vi "ADIS16470 Open.vi"(7 "Buffer Size (0)":u32, 8 "error in":errorcluster, 9 "Initial Calibration Time (4s)":dbl=4.0, 10 "Sychronous Process VI":T1, 11 "Hardware Config":T3={"SPI Clock Rate (Hz)"=2000000.0, "IMU SPI Mode (3)"=enum."Mode 3 (Clk Idle High,Sample on Trailing)", "IMU Reset Pin"=enum."SPI Port CS2", "IMU SPI Bus"=enum."SPI On-Board, CS0", "IMU Data Ready Pin"=enum."SPI Port CS1", "Stall Config"={"Pow2BytesPerRead"=1, "StallTicks"=1000, "CsToSclkTicks"=5}}) -> (0 "error out":errorcluster, 3 "ADIS16470DevRef":T2={"DevStatus"={"status"=FALSE, "code"=0, "source"=""}, "Hardware Config"={"SPI Clock Rate (Hz)"=1000000.0, "IMU SPI Mode (3)"=enum."Mode 3 (Clk Idle High,Sample on Trailing)", "IMU Reset Pin"=enum."SPI Port CS2", "IMU SPI Bus"=enum."SPI On-Board, CS0", "IMU Data Ready Pin"=enum."SPI Port CS1", "Stall Config"={"Pow2BytesPerRead"=255, "StallTicks"=640, "CsToSclkTicks"=5}}, "Calibration Complete"=refnum, "Status Reference"=refnum, "Data Reference"=refnum, "Sychronous Process VI"=refnum, "Cmd FIFO"=refnum, "Source"={"DevStatus"={"status"=FALSE, "code"=0, "source"=""}, "AnalogTriggerMode?"=FALSE, "DigitalMode"={"DIO Channel"=enum."Disabled"}, "AnalogTriggerMode"={"AnalogTriggerIndex"=enum."Trig 0", "OutputType"=enum."InWindow"}}, "Data FIFO"=refnum, "Calibration Time (ms)"=5, "Data Reference"=refnum})   [LabVIEW 2025]
doc: "Open and initialize a session for the ADI 16470 IMU. This calibrates, and then integrates X, Y, and Z angles. Acceleration and other IMU values are not currently surfaced, but are accessible if added to the API. It is advised that you have the robot stationary while being calibrated."
uses:
  <vilib>/Rock Robotics/WPI/ThirdParty/ADI/ADIS16470/Typedef/ADIS16470 Hardware Configuration.ctl
  <vilib>/Rock Robotics/WPI/SPI/WPI_SPIMode.ctl
  <vilib>/Rock Robotics/SystemInterfaces/DIO/FPGA_DIOChannel.ctl
  <vilib>/Rock Robotics/SystemInterfaces/spilib/spi_bus.ctl
  <vilib>/Rock Robotics/WPI/ThirdParty/ADI/ADIS16470/Typedef/ADIS16470 Device Reference.ctl
  <vilib>/Rock Robotics/WPI/ThirdParty/ADI/ADIS16470/Typedef/ADIS16470 Status.ctl
  <vilib>/Rock Robotics/WPI/ThirdParty/ADI/ADIS16470/Typedef/ADIS16470 Data.ctl
  <vilib>/Rock Robotics/WPI/ThirdParty/ADI/ADIS16470/Typedef/ADIS16470 Process.ctl
  <vilib>/Rock Robotics/WPI/ThirdParty/ADI/ADIS16470/Typedef/ADIS16470 Command Type.ctl
  <vilib>/Rock Robotics/SystemInterfaces/CounterEncoderSourceConvertion/FPGA_CounterEncoderSourceConvertionLVSourceType.ctl
  <vilib>/Rock Robotics/SystemInterfaces/DIO/FPGA_DIODigitalSourceChannel.ctl
  <vilib>/Rock Robotics/SystemInterfaces/AnalogTrigger/FPGA_AnalogTriggerIndex.ctl
  <vilib>/Rock Robotics/SystemInterfaces/AnalogTrigger/FPGA_AnalogTriggerOutType.ctl
  <vilib>/Rock Robotics/SystemInterfaces/NetworkCommunication/NetComm_UsageReport_ResourceType.ctl
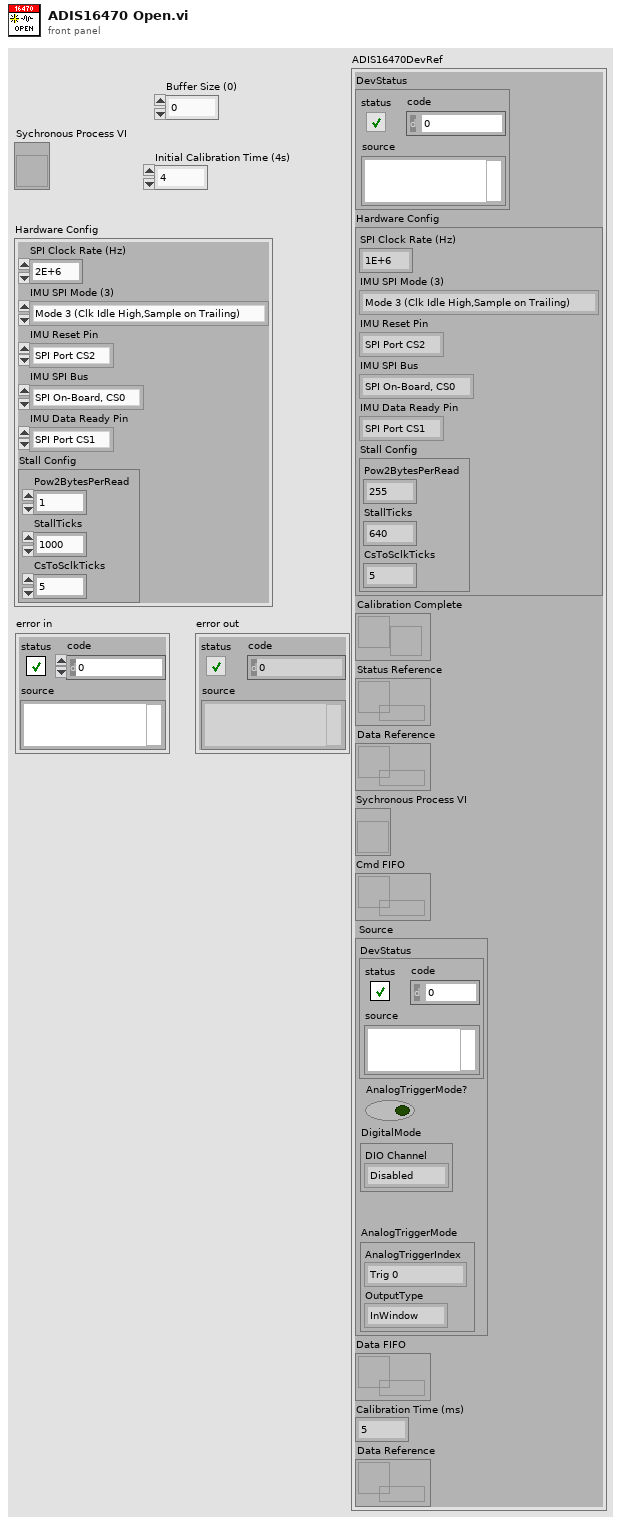
[diagram p1: front panel]
types:
  T1 = typedef "ADIS16470 Process.ctl" = refnum<vi>
  T2 = typedef "ADIS16470 Device Reference.ctl" = cluster{"DevStatus":errorcluster, "Hardware Config":T3, "Calibration Complete":refnum<notifier>, "Status Reference":refnum<data-value>, "Data Reference":refnum<data-value>, "Sychronous Process VI":T1, "Cmd FIFO":refnum<k33>, "Source":T7, "Data FIFO":refnum<k33>, "Calibration Time (ms)":u32, "Data Reference":refnum<data-value>}
  T3 = typedef "ADIS16470 Hardware Configuration.ctl" = cluster{"SPI Clock Rate (Hz)":dbl, "IMU SPI Mode (3)":T4, "IMU Reset Pin":T5, "IMU SPI Bus":T6, "IMU Data Ready Pin":T5, "Stall Config":cluster{"Pow2BytesPerRead":u8, "StallTicks":u16, "CsToSclkTicks":u8}}
  T4 = typedef "WPI_SPIMode.ctl" = enum16{"Mode 0 (Clk Idle Low,Sample on Leading)", "Mode 1 (Clk Idle Low,Sample on Trailing)", "Mode 2 (Clk Idle High,Sample on Leading)", "Mode 3 (Clk Idle High,Sample on Trailing)"}
  T5 = typedef "FPGA_DIOChannel.ctl" = enum8{"DIO 0", "DIO 1", "DIO 2", "DIO 3", "DIO 4", "DIO 5", "DIO 6", "DIO 7", "DIO 8", "DIO 9", "DIO MXP 0", "DIO MXP 1", "DIO MXP 2", "DIO MXP 3", "DIO MXP 4", "DIO MXP 5", "DIO MXP 6", "DIO MXP 7", "DIO MXP 8", "DIO MXP 9", "DIO MXP 10", "DIO MXP 11", "DIO MXP 12", "DIO MXP 13", "DIO MXP 14", "DIO MXP 15", "SPI Port CS1", "SPI Port CS2", "SPI Port CS3", "SPI Port MISO", "SPI Port MOSI", "Invalid"}
  T6 = typedef "spi_bus.ctl" = enum16{"SPI On-Board, CS0", "SPI On-Board, CS1", "SPI On-Board, CS2", "SPI On-Board, CS3", "SPI MXP", "Invalid"}
  T7 = typedef "FPGA_CounterEncoderSourceConvertionLVSourceType.ctl" = cluster{"DevStatus":errorcluster, "AnalogTriggerMode?":bool, "DigitalMode":cluster{"DIO Channel":T8}, "AnalogTriggerMode":cluster{"AnalogTriggerIndex":T9, "OutputType":T10}}
  T8 = typedef "FPGA_DIODigitalSourceChannel.ctl" = enum8{"DIO 0", "DIO 1", "DIO 2", "DIO 3", "DIO 4", "DIO 5", "DIO 6", "DIO 7", "DIO 8", "DIO 9", "DIO MXP 0", "DIO MXP 1", "DIO MXP 2", "DIO MXP 3", "DIO MXP 4", "DIO MXP 5", "DIO MXP 6", "DIO MXP 7", "DIO MXP 8", "DIO MXP 9", "DIO MXP 10", "DIO MXP 11", "DIO MXP 12", "DIO MXP 13", "DIO MXP 14", "DIO MXP 15", "SPI Port CS1", "SPI Port CS2", "SPI Port CS3", "SPI Port MISO", "SPI Port MOSI", "Disabled"}
  T9 = typedef "FPGA_AnalogTriggerIndex.ctl" = enum8{"Trig 0", "Trig 1", "Trig 2", "Trig 3", "Trig 4", "Trig 5", "Trig 6", "Trig 7", "Invalid"}
  T10 = typedef "FPGA_AnalogTriggerOutType.ctl" = enum16{"InWindow", "TriggerState", "Rising", "Falling"}
  T11 = typedef "ADIS16470 Data.ctl" = cluster{"XAngle":dbl, "YAngle":dbl, "ZAngle":dbl}
  T12 = typedef "ADIS16470 Command Type.ctl" = cluster{"Command":enum16{"None", "Reset", "Recalibrate"}, "Data":u32}
  T13 = typedef "ADIS16470 Status.ctl" = cluster{"Calibrated?":bool, "IMU Detected?":bool}
  T14 = typedef "NetComm_UsageReport_ResourceType.ctl" = enum8{"Controller", "Module", "Language", "CANPlugin", "Accelerometer", "ADXL345", "AnalogChannel", "AnalogTrigger", "AnalogTriggerOutput", "CANJaguar", "Compressor", "Counter", "Dashboard", "DigitalInput", "DigitalOutput", "DriverStationCIO", "DriverStationEIO", "DriverStationLCD", "Encoder", "GearTooth", "Gyro", "I2C", "Framework", "Jaguar", "Joystick", "Kinect", "KinectStick", "PIDController", "Preferences", "PWM", "Relay", "RobotDrive", "SerialPort", "Servo", "Solenoid", "SPI", "Task", "Ultrasonic", "Victor", "Button", "Command", "AxisCamera", "PCVideoServer", "SmartDashboard", "Talon", "HiTechnicColorSensor", "HiTechnicAccel", "HiTechnicCompass", "SRF08", "AnalogOutput", "Victor SP", "Talon SRX", "CAN Talon SRX", "ADXL362 Accel", "ADXRS450 Gyro", "Rev SPARK", "Mindsensors SD540", "Digital Filter", "ADIS16448", "PDP", "PCM", "PigeonIMU", "Nidec Brushless", "CTRE CANifier", "CTRE TalonFX", "CTRE Future 1", "CTRE Future 2", "CTRE Future 3", "CTRE Future 4", "CTRE Future 5", "CTRE Future 6", "Linear Filter", "Xbox Controller", "USB Camera", "NavX", "Pixy", "Pixy2", "ScanseSweep", "Shuffleboard", "CAN", "Digilent DMC60", "PWM Victor SPX", "Rev SPARK MAX PWM", "Rev SPARK MAX CAN", "ADIS16470", "PIDController2", "ProfiledPIDController", "Kinematics", "Odometry", "Units", "Trapezoid Profile", "DutyCycle", "Addressable LEDs", "Fusion Venom", "CTRE Future 7", "CTRE Future 8", "CTRE Future 9", "CTRE Future 10", "CTRE Future 11", "CTRE Future 12", "CTRE Future 13", "CTRE Future 14", "Exponential Profile", "PS4 Controller", "Photon Camera", "Photon Pose Estimator", "Path Planner Path", "Path Planner Auto", "Path Finding Command", "Redux Future 1", "Redux Future 2", "Redux Future 3", "Redux Future 4", "Redux Future 5", "Rev SPARK Flex CAN", "Rev SPARK Flex PWM", "LEDPattern", "LinearQuadraticRegulator", "KalmanFilter", "PoseEstimator", "PoseEstimator3d", "LinearSystemLoop", "WPILib_future7", "WPILib_future8", "Rev_ServoHub", "YAMS", "LumenLabs_ConnectorX", "LumenLabs_ConnectorXLED"}
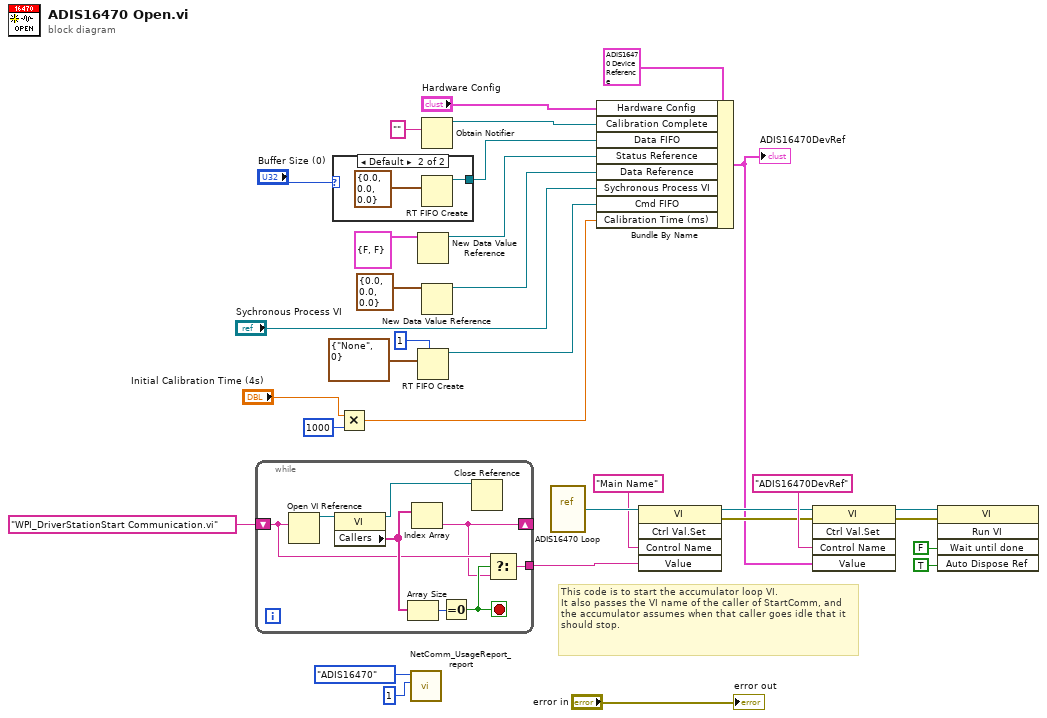
[diagram p0: block diagram]
diagram:
  # "This code is to start the accumulator loop VI.\nIt also passes the VI name of the caller of StartComm, and the accumulator assumes when that caller goes idle that it should stop."
  n1 = while {
    shift-right: [w35] -> _
    shift-left: "WPI_DriverStationStart Communication.vi" -> [w36]
    tunnel: [w34] -> w22
    stop <- w37 stop-if-true
    n2 = Open VI Reference(vi path=w36) -> (vi reference=w40:refnum<vi>)  [unwired: 1 in, 5 out]
    n3 = property class="VI"(reference=w40) -> (reference out=w33:refnum<vi>, "Callers"=w38:string[])  [unwired: 1 in, 1 out]
    n4 = Array Size(array=w38) -> (size(s)=w39:i32)
    n5 = Index Array(array=w38) -> (element=w35:string)  [unwired: 1 in]
    n6 = Equal To 0?(x=w39) -> (x = 0?=w37:bool)
    n7 = Close Reference(reference=w33) -> ()  [unwired: 1 in, 1 out]
    n8 = Select(t=w36, s=w37, f=w35) -> (s? t:f=w34:string)
  }
  n9 = case shown="Default" "Buffer Size (0)" {
    tunnel: [_ w41] -> w15
    frame 0 {
    }
    frame Default {
      n10 = RT FIFO Create(1:T11 {"XAngle"=0.0, "YAngle"=0.0, "ZAngle"=0.0}) -> (8:w41:refnum<k33>)  [unwired: 7 in, 2 out]
    }
  }
  n11 = Multiply(x="Initial Calibration Time (4s)", y=u32 1000 ("size (10)")) -> (x*y=w1:dbl)
  n12 = call <vilib>:"NetComm_UsageReport_report.vi"("Instance Number"=u8 1, "Resource Type"=NetComm_UsageReport_ResourceType."ADIS16470") -> ()  [unwired: 10 in]
  n13 = New Data Value Reference(data value=T13 {"Calibrated?"=FALSE, "IMU Detected?"=FALSE}) -> (data value reference=w9:refnum<data-value>)  [unwired: 1 in, 1 out]
  n14 = RT FIFO Create(1:T12 {"Command"=enum."None", "Data"=0}, 4:u32 1 ("size (10)")) -> (8:w11:refnum<k33>)  [unwired: 6 in, 2 out]
  n15 = Obtain Notifier(notification data type="") -> (notifier out=w17:refnum<notifier>)  [unwired: 3 in, 2 out]
  n16 = New Data Value Reference(data value=T11 {"XAngle"=0.0, "YAngle"=0.0, "ZAngle"=0.0}) -> (data value reference=w8:refnum<data-value>)  [unwired: 1 in, 1 out]
  n17 = vi-ref <vilib>:"ADIS16470 Loop.vi"() -> (w24:refnum<vi>)
  n18 = Bundle By Name(cluster=T2 {"DevStatus"={"status"=FALSE, "code"=0, "source"=""}, "Hardware Config"={"SPI Clock Rate (Hz)"=1000000.0, "IMU SPI Mode (3)"=enum."Mode 3 (Clk Idle High,Sample on Trailing)", "IMU Reset Pin"=enum."SPI Port CS2", "IMU SPI Bus"=enum."SPI On-Board, CS0", "IMU Data Ready Pin"=enum."SPI Port CS1", "Stall Config"={"Pow2BytesPerRead"=255, "StallTicks"=640, "CsToSclkTicks"=5}}, "Calibration Complete"=refnum, "Status Reference"=refnum, "Data Reference"=refnum, "Sychronous Process VI"=refnum, "Cmd FIFO"=refnum, "Source"={"DevStatus"={"status"=FALSE, "code"=0, "source"=""}, "AnalogTriggerMode?"=FALSE, "DigitalMode"={"DIO Channel"=enum."Disabled"}, "AnalogTriggerMode"={"AnalogTriggerIndex"=enum."Trig 0", "OutputType"=enum."InWindow"}}, "Data FIFO"=refnum, "Calibration Time (ms)"=5, "Data Reference"=refnum} ("ADIS16470DevRef"), "Hardware Config"="Hardware Config", "Calibration Complete"=w17, "Data FIFO"=w15, "Status Reference"=w9, "Data Reference"=w8, "Sychronous Process VI"="Sychronous Process VI", "Cmd FIFO"=w11, "Calibration Time (ms)"=w1) -> (w18:T2)
  "ADIS16470DevRef" <- w18
  n19 = invoke class="VI" method="Ctrl Val.Set"(reference=w24, "Control Name"="Main Name", "Value"=w22) -> (reference out=w21:refnum<vi>, error out=w26:errorcluster)  [unwired: 2 in, 3 out]
  n20 = invoke class="VI" method="Ctrl Val.Set"(reference=w21, error in=w26, "Control Name"="ADIS16470DevRef", "Value"=w18) -> (reference out=w5:refnum<vi>, error out=w4:errorcluster)  [unwired: 1 in, 3 out]
  n21 = invoke class="VI" method="Run VI"(reference=w5, error in=w4, "Wait until done"=FALSE ("Wait Until Done"), "Auto Dispose Ref"=TRUE ("Auto Dispose Reference")) -> ()  [unwired: 1 in, 5 out]
  "error out" <- "error in"
